vi "save AlarmCode Xml.vi"(8 "error in (no error)":errorcluster, 10 "project":T1, 11 "XML File Path":path caption="XML文件路径") -> (0 "error out":errorcluster)   [LabVIEW 2022 SP3, in "opSignIn.lvlib"]
uses:
  opSignIn.lvlib
  <vilib>/Utility/xml.llb/Write to XML File(string).vi
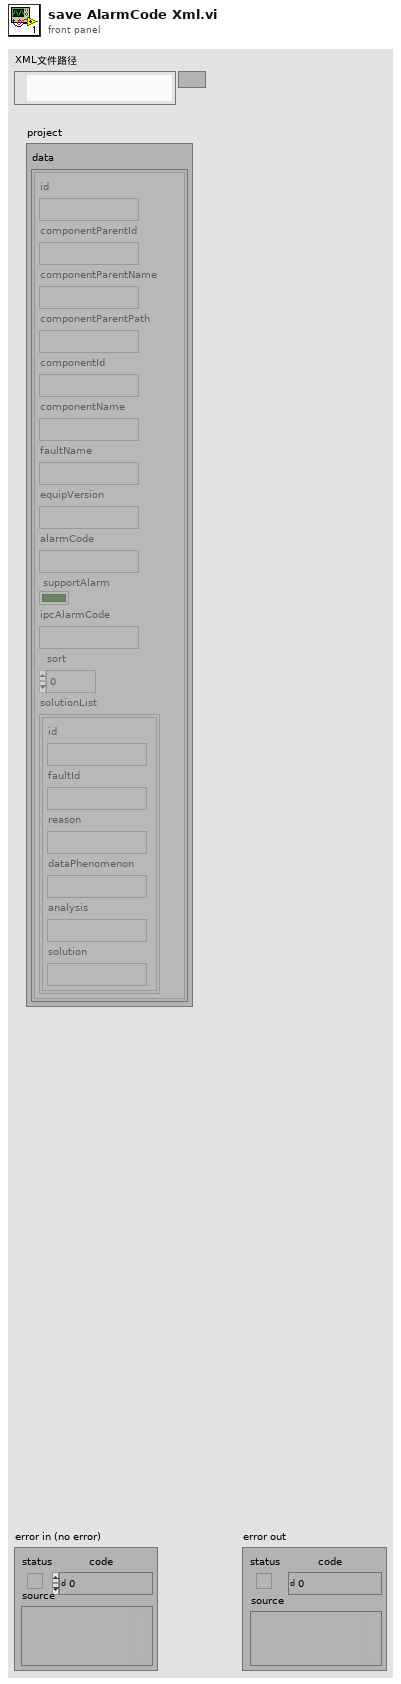
[diagram p1: front panel]
types:
  T1 = typedef "opSignIn.lvlib/报警格式.ctl" = cluster{"data":T2[]}
  T2 = typedef "opSignIn.lvlib/元素.ctl" = cluster{"id":string, "componentParentId":string, "componentParentName":string, "componentParentPath":string, "componentId":string, "componentName":string, "faultName":string, "equipVersion":string, "alarmCode":string, "supportAlarm":bool, "ipcAlarmCode":string, "sort":dbl, "solutionList":cluster{"id":string, "faultId":string, "reason":string, "dataPhenomenon":string, "analysis":string, "solution":string}[]}
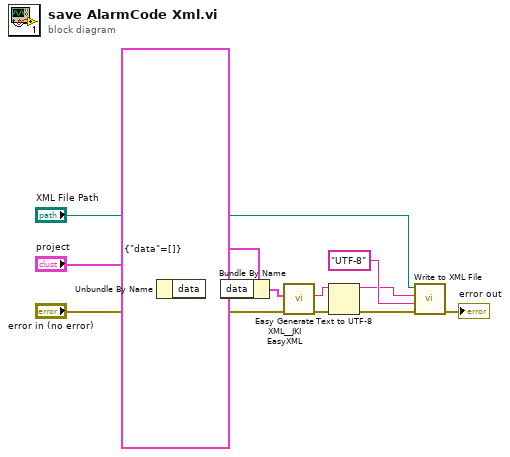
[diagram p0: block diagram]
diagram:
  n1 = Unbundle By Name("project") -> ("data"=w7:T2[])
  n2 = Bundle By Name(cluster=T1 {"data"=[]} ("project"), "data"=w7) -> (w10:T1)
  n3 = call <vilib>:"Easy Generate XML__JKI EasyXML.vi"("error in (no error)"="error in (no error)", "LabVIEW Data"=w10) -> ("error out"=w5:errorcluster, "XML String"=w11:string)  [unwired: 8 in]
  n4 = Text to UTF-8(8:w5, 11:w11) -> (0:w4:errorcluster, 3:w9:string)  [unwired: 1 in]
  n5 = call-poly <vilib>:"Write to XML File.vi"("error in (no error)"=w4, "XML Encoding"="UTF-8", "XML Input"=w9, "XML File Path"="XML File Path") -> ("error out"=→"error out":errorcluster)  [unwired: 5 in, 2 out]
